vi "Position Horizontal Splitter.vi"(8 "error in (no error)":errorcluster, 11 "This VI":refnum<vi>) -> (0 "error out":errorcluster)   [LabVIEW 2014]
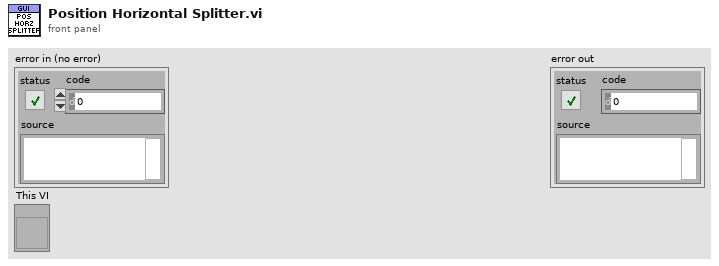
[diagram p1: front panel]
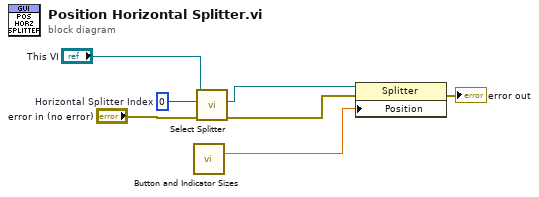
[diagram p0: block diagram]
diagram:
  w5 = 0  # Horizontal Splitter Index
  n1 = call "Button and Indicator Sizes.vi"() -> ("Button Height"=w2:dbl)  [unwired: 11 in, 4 out]
  n2 = call "Select Splitter.vi"("error in (no error)"="error in (no error)", "Pane Index"=w5, "This VI"="This VI") -> ("error out"=w3:errorcluster, "Splitter"=w4:refnum<vi>)  [unwired: 6 in, 1 out]
  n3 = property class="Splitter"(reference=w4, error in=w3, "Position"=w2) -> (error out=→"error out":errorcluster)  [unwired: 1 out]
